vi "ExtractModuleID.vi"(7 "ModuleType":string="AcPwr", 8 "error in":errorcluster, 10 "Module List":variant, 11 "Test.lvclass In":refnum<class "Test.lvclass">) -> (0 "Error Out":errorcluster, 1 "ModuleIDs":i32, 2 "String":string, 3 "Test.lvclass Out":refnum<class "Test.lvclass">, 4 "Variant Output(Module List for Debugging)":variant)   [LabVIEW 2018, in "Test.lvclass"]
doc: "Parses the incoming message variant and determines if the message should be sent to all clones ( specific to a given module) or a specific clone in that module."
uses:
  Test.lvclass
  Test.lvclass/Test.ctl
  Accessors/Read ErrorSeverity.vi
  Accessors/Read ModuleIDs.vi
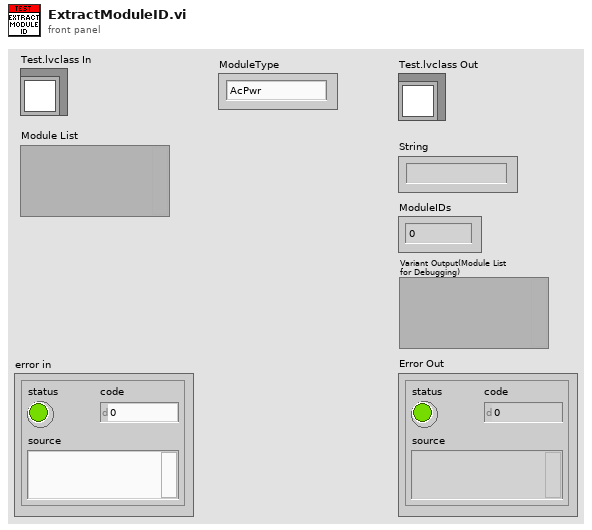
[diagram p1: front panel]
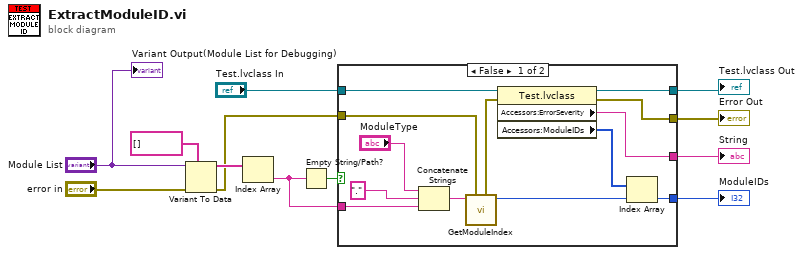
[diagram p0: block diagram]
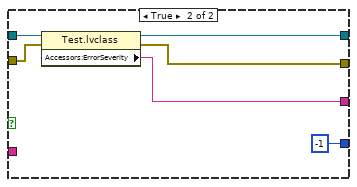
[diagram p2: hidden frame]
diagram:
  n1 = Variant To Data(error in="error in", type=string[] [], Variant="Module List") -> (data=w12:string[], error out=w10:errorcluster)
  n2 = Index Array(array=w12) -> (element=w8:string)  [unwired: 1 in]
  n3 = Empty String/Path?(string/path=w8) -> (empty?=w2:bool)
  n4 = case shown="False" w2 {
    tunnel: w10 -> [w25 w31]
    tunnel: w8 -> [w21 _]
    tunnel: "Test.lvclass In" -> [w19 w30]
    tunnel: [w18 w29] -> w6
    tunnel: [w17 w26] -> w5
    tunnel: [w14 -1 ("f")] -> w4
    tunnel: [w15 w28] -> w3
    frame False {
      n5 = Concatenate Strings("ModuleType", "." ("string"), w21) -> (w22:string)
      n6 = call "GetModuleIndex.vi"("Error In"=w25, "ModuleType"=w22) -> ("ModuleIndex"=w13:i32, "Error"=w16:errorcluster)  [unwired: 8 in]
      n7 = property class="Test.lvclass"(reference=w19, error in=w16) -> (reference out=w18:refnum<class "Test.lvclass">, error out=w17:errorcluster, "Accessors:ErrorSeverity"=w15:string, "Accessors:ModuleIDs"=w20:i32[])
      n8 = Index Array(array=w20, index=w13) -> (element=w14:i32)
    }
    frame True {
      n9 = property class="Test.lvclass"(reference=w30, error in=w31) -> (reference out=w29:refnum<class "Test.lvclass">, error out=w26:errorcluster, "Accessors:ErrorSeverity"=w28:string)
    }
  }
  "Error Out" <- w5
  "ModuleIDs" <- w4
  "Test.lvclass Out" <- w6
  "String" <- w3
  "Variant Output(Module List for Debugging)" <- "Module List"
